vi "Agilent VNA Set Channel Display.vi"(6 "Channel":i32=1 min=1 max=99 step=1, 7 "Agilent VNA":T1, 8 "error in (no error)":errorcluster, 11 "VISA Resource Name":refnum<visa-resource-name>) -> (0 "error out":errorcluster, 3 "dup VISA Resource Name":refnum<visa-resource-name>)   [LabVIEW 2011]
uses:
  TypeDefs/Agilent VNA Display.ctl
  TypeDefs/Agilent VNA Instrument Info.ctl
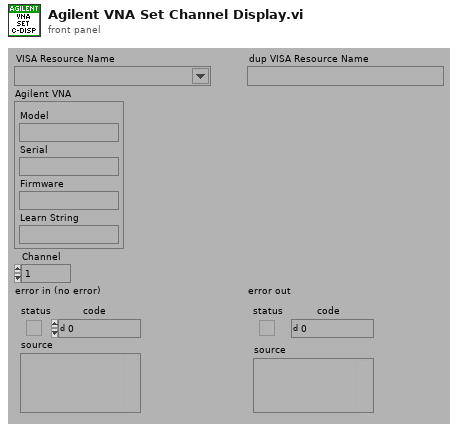
[diagram p1: front panel]
types:
  T1 = typedef "Agilent VNA Instrument Info.ctl" = cluster{"Model":string, "Serial":string, "Firmware":string, "Learn String":string}
  T2 = typedef "Agilent VNA Model.ctl" = enum16{"Not Supported", "8510X", "8719X", "8720X", "8722X", "8753X", "ENA", "PNA", "Field Fox"}
  T3 = typedef "Agilent VNA Display.ctl" = enum16{"D1", "D12", "D1_2", "D112", "D1_1_2", "D123", "D1_2_3", "D12_33", "D11_23", "D13_23", "D12_13", "D1234", "D1_2_3_4", "D12_34", "D123_456", "D12_34_56", "D1234_5678", "D12_34_56_78", "D123_456_789", "D123__ABC", "D1234__9ABC", "D1234__DEFG"}
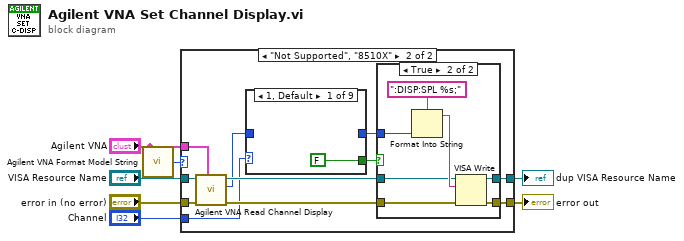
[diagram p0: block diagram]
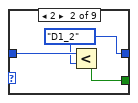
[diagram p4: hidden frame]
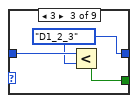
[diagram p5: hidden frame]
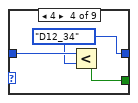
[diagram p6: hidden frame]
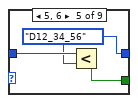
[diagram p7: hidden frame]
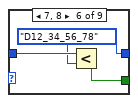
[diagram p8: hidden frame]
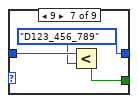
[diagram p9: hidden frame]
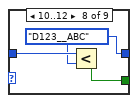
[diagram p10: hidden frame]
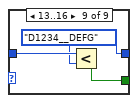
[diagram p11: hidden frame]
diagram:
  n1 = call "Agilent VNA Format Model String.vi"("Model"="Agilent VNA") -> ("Model"=w3:T2)
  n2 = case shown="\"E5070B\", \"E5071B\"" w3 {
    tunnel: "VISA Resource Name" -> [w9 w17]
    tunnel: "error in (no error)" -> [w8 w18]
    tunnel: [w9 w20] -> w5
    tunnel: [w8 w19] -> w4
    tunnel: "Channel" -> [_ w14]
    tunnel: "Agilent VNA" -> [_ w11]
    frame Default {
    }
    frame "Not Supported", "8510X" {
      n3 = call "Agilent VNA Read Channel Display.vi"("Agilent VNA"=w11, "error in (no error)"=w18, "VISA Resource Name"=w17) -> ("error out"=w15:errorcluster, "Display"=w13:T3, "dup VISA Resource Name"=w16:refnum<visa-resource-name>)  [unwired: 6 in]
      n4 = case shown="1, Default" w14 {
        tunnel: w13 -> [_ w33 w36 w39 w42 w45 w48 w51 w54]
        tunnel: [FALSE w32 w35 w38 w41 w44 w47 w50 w53] -> w10
        tunnel: [_ w31 w34 w37 w40 w43 w46 w49 w52] -> w12
        frame 1, Default {
        }
        frame 2 {
          w31 = Agilent_VNA_Display."D1_2" ("y")
          n5 = Less?(x=w33, y=w31) -> (x < y?=w32:bool)
        }
        frame 3 {
          w34 = Agilent_VNA_Display."D1_2_3" ("y")
          n6 = Less?(x=w36, y=w34) -> (x < y?=w35:bool)
        }
        frame 4 {
          w37 = Agilent_VNA_Display."D12_34" ("y")
          n7 = Less?(x=w39, y=w37) -> (x < y?=w38:bool)
        }
        frame 5, 6 {
          w40 = Agilent_VNA_Display."D12_34_56" ("y")
          n8 = Less?(x=w42, y=w40) -> (x < y?=w41:bool)
        }
        frame 7, 8 {
          w43 = Agilent_VNA_Display."D12_34_56_78" ("y")
          n9 = Less?(x=w45, y=w43) -> (x < y?=w44:bool)
        }
        frame 9 {
          w46 = Agilent_VNA_Display."D123_456_789" ("y")
          n10 = Less?(x=w48, y=w46) -> (x < y?=w47:bool)
        }
        frame 10..12 {
          w49 = Agilent_VNA_Display."D123__ABC" ("y")
          n11 = Less?(x=w51, y=w49) -> (x < y?=w50:bool)
        }
        frame 13..16 {
          w52 = Agilent_VNA_Display."D1234__DEFG" ("y")
          n12 = Less?(x=w54, y=w52) -> (x < y?=w53:bool)
        }
      }
      n13 = case shown="True" w10 {
        tunnel: [w22 w29] -> w20
        tunnel: [w21 w28] -> w19
        tunnel: w16 -> [w22 w25]
        tunnel: w15 -> [w21 w24]
        tunnel: w12 -> [_ w23]
        frame False {
        }
        frame True {
          n14 = Format Into String(format string=":DISP:SPL %s;" ("write buffer"), w23) -> (resulting string=w26:string)  [unwired: 2 in, 1 out]
          n15 = VISA Write(VISA resource name=w25, write buffer=w26, error in (no error)=w24) -> (VISA resource name out=w29:refnum<visa-resource-name>, error out=w28:errorcluster)  [unwired: 1 out]
        }
      }
    }
  }
  "dup VISA Resource Name" <- w5
  "error out" <- w4
